vi "GetProcessNotifierFromRef.vi"(8 "error in (no error)":errorcluster, 10 "Process VI Refnum":refnum<vi>, 11 "SMO":refnum<class "SMO.lvclass">) -> (0 "error out":errorcluster, 2 "Sync Notifier":refnum<notifier>, 3 "SMO out":refnum<class "SMO.lvclass">)   [LabVIEW 2013, in "SMO.lvclass"]
doc: "This method will lookup (and return) the instance reference of <b>Process Name</b>.\n\n---------------------------------------------------------------\nJKI State Machine Objects™\nhttp://jki.net/state-machine-objects/\nCopyright (C) 2005-2015, JKI <info@jki.net>\nALL RIGHTS RESERVED"
uses:
  SMO.lvclass
  SMO.lvclass/SMO.ctl
panel:
  # "For instructions on how to use the JKI State Machine Objects, examples and video tutorials, visit:\nhttp://jki.net/state-machine-objects/\n\nJKI State Machine Objects™\nhttp://jki.net/state-machine-objects/\nCopyright (C) 2005-2015, JKI <info@jki.net>\nALL RIGHTS RESERVED"
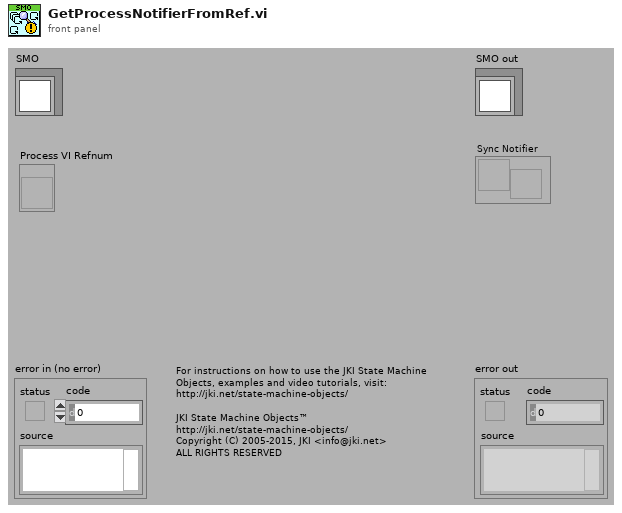
[diagram p1: front panel]
types:
  T1 = typedef "SMO.lvclass/PrivateData--Ref.ctl" = refnum<data-value>
  T2 = typedef "SMO.lvclass/PrivateData--Cluster.ctl" = cluster{"Parent Call":T3, "Registered Processes":T4[], "Sync Notifier":refnum<notifier>, "Process Error Notifier":refnum<notifier>, "Protected Events":T5, "Public Events":T6, "SMO State":T7, "[Dependencies]":T8[], "[Attributes]":refnum<class "Attribute.lvclass">[], "Launcher Close":refnum<notifier>}
  T3 = typedef "SMO.lvclass/Parent Call--Enum.ctl" = enum16{"Allows parent to run", "Does not request parent to run"}
  T4 = typedef "SMO.lvclass/RegisteredProcessData--Cluster.ctl" = cluster{"Name":string, "Static VI Ref":refnum<vi>, "Running":bool, "NotifierRef":u32}
  T5 = typedef "SMO.lvclass/Protected Events.ctl" = cluster{"StopProcesses":refnum<user-event>, "AbortProcesses":refnum<user-event>, "Config Changed":refnum<user-event>}
  T6 = typedef "SMO.lvclass/Public Events.ctl" = cluster{"Error":refnum<user-event>, "State":refnum<user-event>}
  T7 = typedef "SMO.lvclass/SMOState --Enum.ctl" = enum16{"unknown", "Created", "Started", "Stopped"}
  T8 = typedef "SMO.lvclass/SMO Dependency--Cluster.ctl" = cluster{"Dependency":refnum<class "SMO.lvclass">, "Level":string}
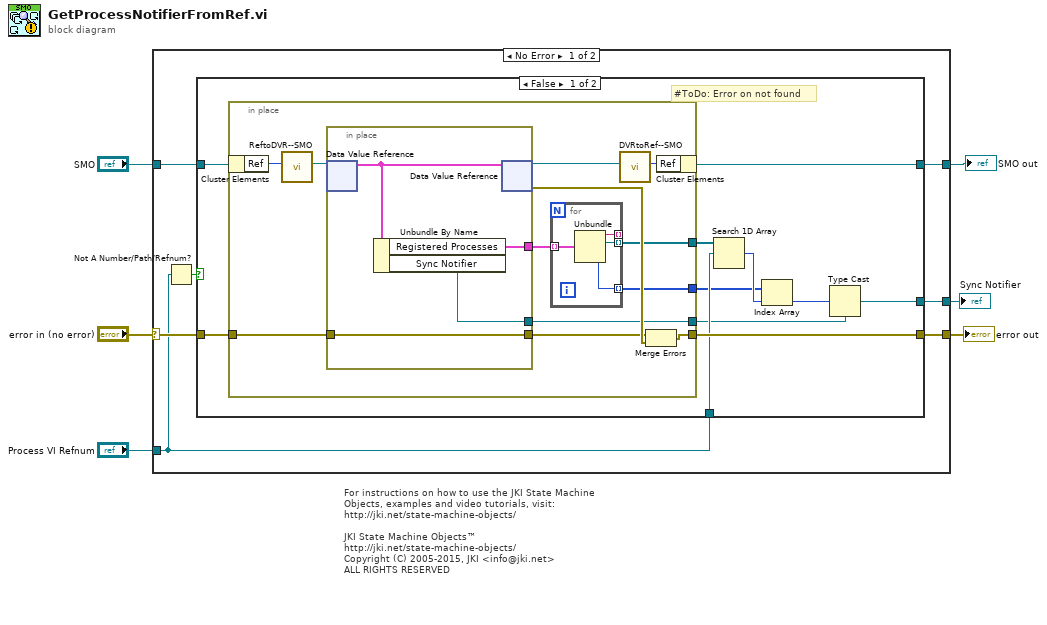
[diagram p0: block diagram]
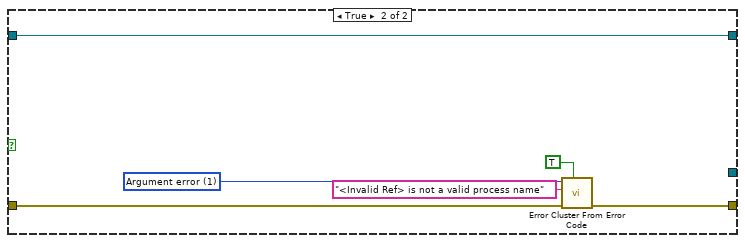
[diagram p2: hidden frame]
diagram:
  # "For instructions on how to use the JKI State Machine Objects, examples and video tutorials, visit:\nhttp://jki.net/state-machine-objects/\n\nJKI State Machine Objects™\nhttp://jki.net/state-machine-objects/\nCopyright (C) 2005-2015, JKI <info@jki.net>\nALL RIGHTS RESERVED"
  n1 = case shown="No Error" "error in (no error)" {
    selector: "error in (no error)" -> [w12 w52]
    tunnel: [w11 w52] -> w2
    tunnel: [w10 w51] -> w3
    tunnel: "SMO" -> [w13 w51]
    tunnel: [w9 _] -> w1
    tunnel: "Process VI Refnum" -> [w7 _]
    frame No Error {
      n2 = Not A Number/Path/Refnum?(number/path/refnum=w7) -> (NaN/Path/Refnum?=w8:bool)
      n3 = case shown="False" w8 {
        tunnel: w13 -> [w24 w50]
        tunnel: w12 -> [w23 w48]
        tunnel: [w22 w47] -> w11
        tunnel: [w21 w50] -> w10
        tunnel: [w15 _] -> w9
        tunnel: w7 -> [w20 _]
        frame False {
          # "#ToDo: Error on not found"
          n4 = in-place {
            in-place-border: w23 -> [w36]
            in-place-border: [w33] -> w22
            in-place-border: [w31] -> w18
            in-place-border: [w26] -> w17
            in-place-border: [w25] -> w14
            n5 = in-place-cluster #1(w24) -> ("Ref"=w28:u32)
            n6 = call "ReftoDVR--SMO.vi"("Ref"=w28) -> ("Ref"=w27:T1)  [unwired: 10 in]
            n7 = in-place {
              in-place-border: w36 -> [w43]
              in-place-border: [w43] -> w34
              in-place-border: [w42] -> w32
              in-place-border: [w41] -> w25
              n8 = in-place-dvr #2(w27) -> (w44:T2)  [unwired: 1 out]
              n9 = Unbundle By Name(w44) -> ("Registered Processes"=w42:T4[], "Sync Notifier"=w41:refnum<notifier>)
              n10 = in-place-dvr #2(w44) -> (w30:T1, w35:errorcluster)
            }
            n11 = for {
              tunnel: w32 -> [w40] mode=indexing
              tunnel: [w39] -> _ mode=indexing
              tunnel: [w38] -> w31 mode=indexing
              tunnel: [w37] -> w26 mode=indexing
              n12 = Unbundle(w40) -> ("Name"=w39:string, "Static VI Ref"=w38:refnum<vi>, "NotifierRef"=w37:u32)  [unwired: 1 out]
            }
            n13 = call "DVRtoRef--SMO.vi"("Ref"=w30) -> ("Ref"=w29:u32)  [unwired: 10 in]
            n14 = Merge Errors(w34, w35) -> (w33:errorcluster)
            n15 = in-place-cluster #1("Ref"=w29) -> (w21:refnum<class "SMO.lvclass">)
          }
          n16 = Search 1D Array(1D array=w18, element=w20) -> (index of element=w19:i32)  [unwired: 1 in]
          n17 = Index Array(array=w17, index=w19) -> (element=w16:u32)
          n18 = Type Cast(type=w14, x=w16) -> (*(type *) &x=w15:refnum<notifier>)
        }
        frame True {
          w49 = 1 items=["No error", "Argument error", "Memory is full", "Out of zone", "End of file", "File already open", "Generic file I/O error", "File not found", "File permission error", "Disk is full", "Duplicate path", "Too many files open", "System feature not enabled", "Resource file not found", "Cannot add resource", "Resource not found", "Image not found", "Image memory error", "Pen does not exist", "Config type invalid", "Config token not found", "Config parse error", "Config memory error", "Bad external code format", "Bad external code offset", "External code not present", "Null window", "Destroy window error", "Null menu", "Print aborted", "Bad print record", "Print driver error", "Windows error during printing", "Memory error during printing", "Print dialog error", "Generic print error", "Invalid device refnum", "Device not found", "Device parameter error", "Device unit error", "Cannot open device", "Device call aborted", "Generic error", "Cancelled by user", "Object ID too low", "Object ID too high", "Object not in heap", "Unknown heap", "Unknown object (invalid DefProc)", "Unknown object (DefProc not in table)", "Message out of range", "Invalid (null) method", "Unknown message", "Manager call not supported", "Bad address", "Network operation in progress", "Network operation timed out", "Connection is busy", "Network attribute not supported", "Network error", "Address in use", "System out of memory", "Connection aborted", "Connection refused", "Not connected", "Already connected", "Connection closed", "Initialization error (interapplication manager)", "Bad occurrence", "Wait on unbound occurrence handler", "Occurrence queue overflow", "Datalog type conflict", "Unused", "Unrecognized type (interapplication manager)", "Memory corrupt", "Failed to make temporary DLL", "Old CIN version", "Drag socket not found", "Failed to load drop-object", "Failed to register OLE object", "Failed to release OLE object", "Format specifier type mismatch", "Unknown format specifier", "Too few format specifiers", "Too many format specifiers", "Scan failed", "Newer CIN version", "Error converting to variant", "Runtime menu error", "Password tampered", "Variant attribute not found", "Incompatible variant data type", "Event data is not available", "Event Store is not present", "Occurrence is not found", "Event Queue is not created", "Event info is not available", "Refnum passed is NULL", "Error retrieving Class GUID", "Error retrieving CoClass GUID", "Error retrieving TypeLib GUID.", "Bad built application magic bytes.", "Specific driver is different from the specific driver associated with the Logical Name.", "There is no session opened to the class driver.", "Max Error", "MAX - Error with config objects", "MAX - Error loading configuration", "MAX - Group not supported"]
          n19 = call <vilib>:"Error Cluster From Error Code.vi"("show call chain? (False)"=TRUE, "error in (no error)"=w48, "error message (\"\")"="<Invalid Ref> is not a valid process name" ("error message (\"\")"), "error code (0)"=w49) -> ("error out"=w47:errorcluster)  [unwired: 5 in]
        }
      }
    }
    frame Error {
    }
  }
  "error out" <- w2
  "SMO out" <- w3
  "Sync Notifier" <- w1
